vi "init print.vi"(9 "error in":errorcluster) -> (1 "error in 2":errorcluster, 2 "Boolean":bool)   [LabVIEW 2009]
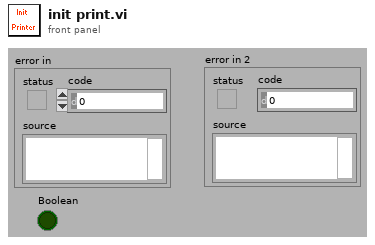
[diagram p1: front panel]
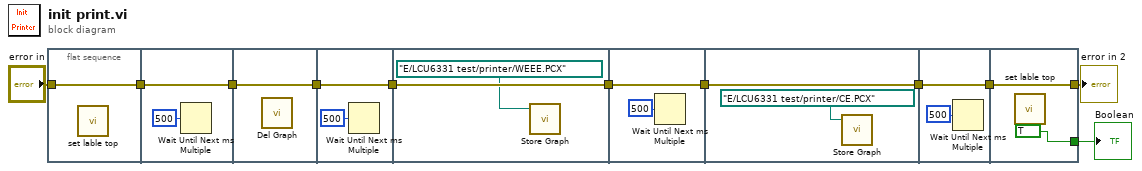
[diagram p0: block diagram]
diagram:
  n1 = flat-sequence {
    tunnel: "error in" -> [w12]
    tunnel: [w12] -> w9
    tunnel: w9 -> [w14]
    tunnel: [w14] -> w8
    tunnel: [w15] -> w7
    tunnel: w8 -> [w15]
    tunnel: w7 -> [w17]
    tunnel: [w17] -> w6
    tunnel: w6 -> [w19]
    tunnel: [w19] -> w3
    tunnel: w3 -> [w21]
    tunnel: [w21] -> w2
    tunnel: w2 -> [w23]
    tunnel: [w23] -> w1
    tunnel: w1 -> [w25]
    tunnel: [w25] -> w5
    tunnel: [w27] -> w10
    tunnel: w5 -> [w27]
    tunnel: [TRUE] -> w4
    frame #0 {
      n2 = call "set lable top.vi"() -> ()  [unwired: 1 out]
    }
    frame #1 {
      n3 = Wait Until Next ms Multiple(millisecond multiple=u32 500) -> ()  [unwired: 1 out]
    }
    frame #2 {
      n4 = call "Del Graph.vi"() -> ()  [unwired: 1 in, 5 out]
    }
    frame #3 {
      n5 = Wait Until Next ms Multiple(millisecond multiple=u32 500) -> ()  [unwired: 1 out]
    }
    frame #4 {
      n6 = call "Store Graph.vi"("file (use dialog)"=path "E:/LCU6331 test/printer/WEEE.PCX") -> ()  [unwired: 5 out]
    }
    frame #5 {
      n7 = Wait Until Next ms Multiple(millisecond multiple=u32 500) -> ()  [unwired: 1 out]
    }
    frame #6 {
      n8 = call "Store Graph.vi"("file (use dialog)"=path "E:/LCU6331 test/printer/CE.PCX") -> ()  [unwired: 5 out]
    }
    frame #7 {
      n9 = Wait Until Next ms Multiple(millisecond multiple=u32 500) -> ()  [unwired: 1 out]
    }
    frame #8 {
      n10 = call "set lable top.vi"() -> ()  [unwired: 1 out]
    }
  }
  "error in 2" <- w10
  "Boolean" <- w4
